vi "Datasheet Format Property Name.vi"(5 "String with \\r or \\n":string) -> (2 "String without \\r or \\n":string)   [LabVIEW 2011]
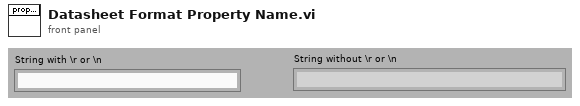
[diagram p1: front panel]
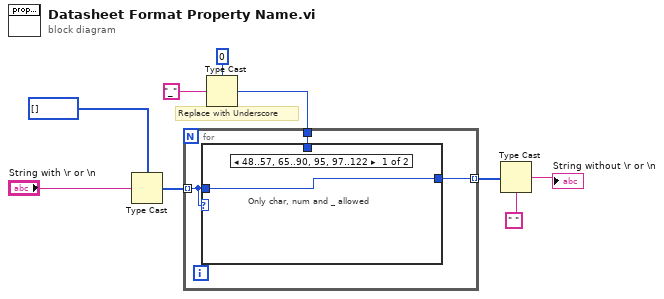
[diagram p0: block diagram]
diagram:
  # "Replace with Underscore"
  n1 = Type Cast(type=u8[] [], x="String with \\r or \\n") -> (*(type *) &x=w7:u8[])
  n2 = Type Cast(type=u8 0, x="_") -> (*(type *) &x=w1:u8)
  n3 = for {
    tunnel: w7 -> [w10] mode=indexing
    tunnel: [w12] -> w6 mode=indexing
    tunnel: w1 -> [w11]
    n4 = case shown="48..57, 65..90, 95, 97..122" w10 {
      tunnel: [w13 w14] -> w12
      tunnel: w11 -> [_ w14]
      tunnel: w10 -> [w13 _]
      frame 48..57, 65..90, 95, 97..122 {
        # "Only char, num and _ allowed"
      }
      frame Default {
      }
    }
  }
  n5 = Type Cast(type=" ", x=w6) -> (*(type *) &x=→"String without \\r or \\n":string)
